vi "Autorange path verification.vi"() -> ()   [LabVIEW 2016]
uses:
  <instrlib>/Zurich Instruments LabOne/Public/ziTypeHandle.ctl
  <vilib>/regexp/Match Regular Expression.xnode
  <instrlib>/Zurich Instruments LabOne/Zurich Instruments LabOne.lvlib
panel:
  out "Path Out":string
  out "Handle Out":T1 {"Handle" format="0x%08x"; "Conn" format="0x%08x"}
  in  "Handle In":T1 {"Handle" format="0x%08x"; "Conn" format="0x%08x"}
  out "concatenated string":string
  out "x >= 0?":bool
  in  "Path 3":string="sigins/0/autorange"
  out "Coerced to new path":string
  in  "Path 2":string="sigins/0/autorange"
  in  "error in (no error) 2":errorcluster
  out "error out 2":errorcluster
  out "error out":errorcluster
  in  "error in (no error)":errorcluster
  in  "Path":string="sigins/0/autorange"
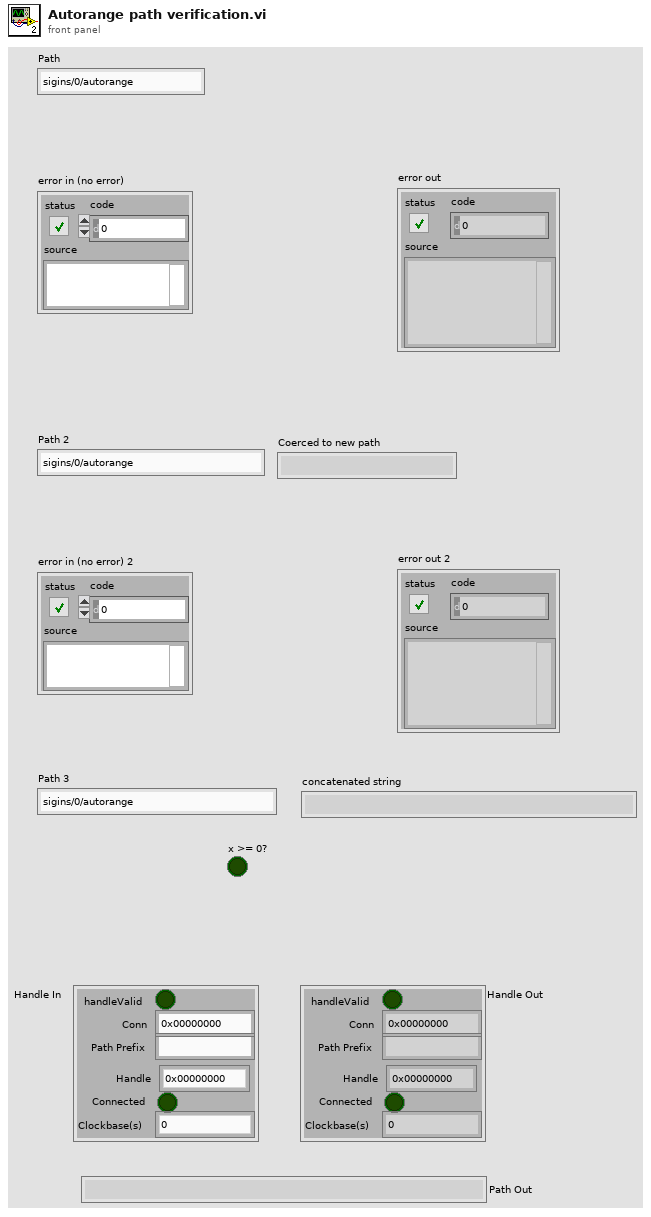
[diagram p1: front panel]
types:
  T1 = typedef "Zurich Instruments LabOne.lvlib/ziTypeHandle.ctl" = cluster{"handleValid":bool, "Conn":u64, "Path Prefix":string, "Handle":u64, "Connected":bool, "Clockbase(s)":dbl}
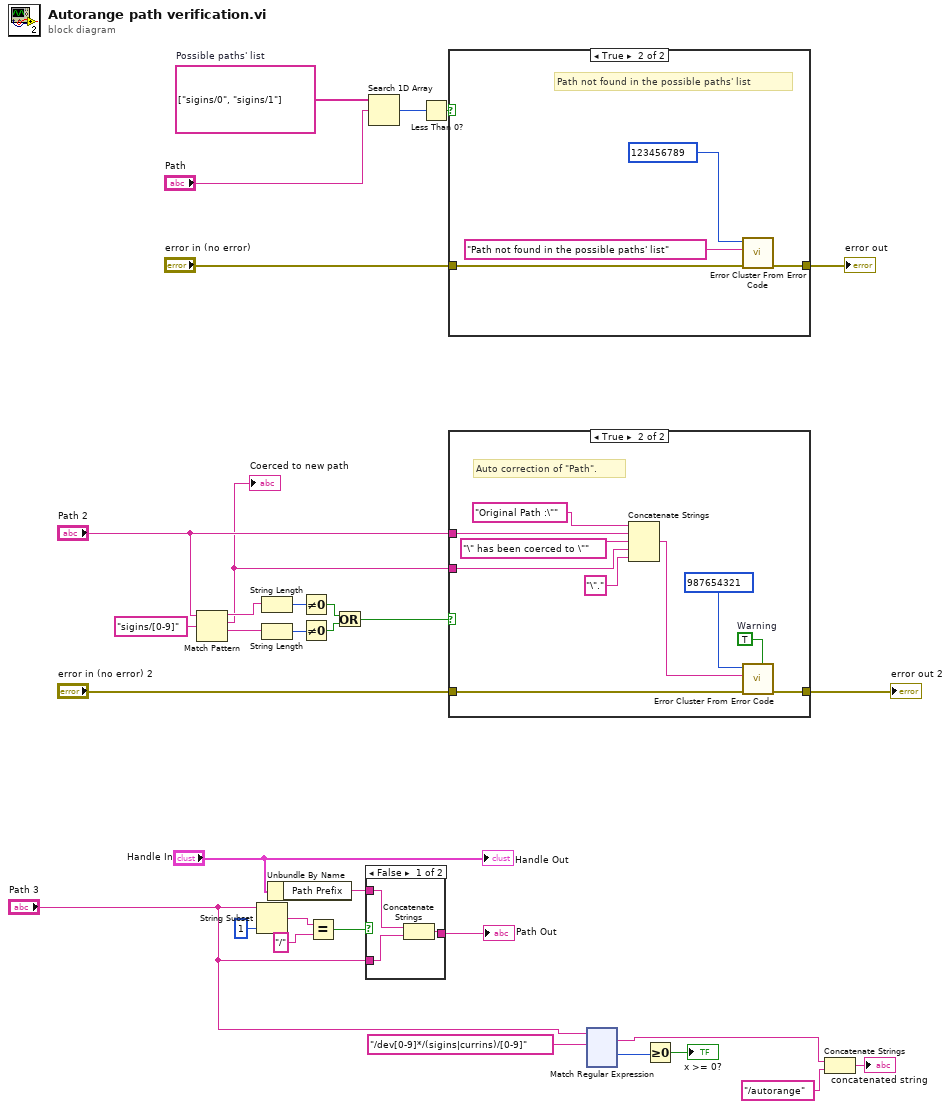
[diagram p0: block diagram]
diagram:
  w32 = string[] ["sigins/0", "sigins/1"]  # Possible paths' list
  n1 = Match Pattern(string="Path 2", regular expression="sigins/[0-9]") -> (before substring=w23:string, match substring=w16:string, after substring=w24:string)  [unwired: 1 in, 1 out]
  "Coerced to new path" <- w16
  n2 = String Subset(string="Path 3", length (rest)=1 ("length (rest)")) -> (substring=w7:string)  [unwired: 1 out]
  n3 = String Length(string=w23) -> (length=w22:i32)
  n4 = String Length(string=w24) -> (length=w21:i32)
  n5 = Unbundle By Name("Handle In") -> ("Path Prefix"=w5:string)
  n6 = Not Equal To 0?(x=w22) -> (x != 0?=w19:bool)
  n7 = Not Equal To 0?(x=w21) -> (x != 0?=w20:bool)
  n8 = Equal?(x=w7, y="/") -> (x = y?=w9:bool)
  n9 = Or(x=w19, y=w20) -> (x .or. y?=w18:bool)
  n10 = case shown="False" w9 {
    tunnel: w5 -> [w33 _]
    tunnel: [w35 w36] -> w3
    tunnel: "Path 3" -> [w34 w36]
    frame False {
      n11 = Concatenate Strings(w33, w34) -> (w35:string)
    }
    frame True {
    }
  }
  "Path Out" <- w3
  n12 = Search 1D Array(1D array=w32, element="Path") -> (index of element=w30:i32)  [unwired: 1 in]
  n13 = Less Than 0?(x=w30) -> (x < 0?=w29:bool)
  n14 = case shown="True" w29 {
    tunnel: "error in (no error)" -> [w37 w41]
    tunnel: [w37 w40] -> w27
    frame False {
    }
    frame True {
      # "Path not found in the possible paths' list"
      n15 = call <vilib>:"Error Cluster From Error Code.vi"("error in (no error)"=w41, "error message (\"\")"="Path not found in the possible paths' list" ("error message (\"\")"), "error code (0)"=123456789) -> ("error out"=w40:errorcluster)  [unwired: 6 in]
    }
  }
  "error out" <- w27
  n16 = case shown="True" w18 {
    tunnel: "error in (no error) 2" -> [w42 w52]
    tunnel: [w42 w51] -> w12
    tunnel: "Path 2" -> [_ w47]
    tunnel: w16 -> [_ w45]
    frame False {
    }
    frame True {
      w49 = TRUE  # Warning
      # "Auto correction of \"Path\"."
      n17 = Concatenate Strings("Original Path :\"", w47, "\" has been coerced to \"" ("string"), w45, "\"." ("string")) -> (w43:string)
      n18 = call <vilib>:"Error Cluster From Error Code.vi"("is warning? (False)"=w49, "error in (no error)"=w52, "error message (\"\")"=w43, "error code (0)"=987654321) -> ("error out"=w51:errorcluster)  [unwired: 5 in]
    }
  }
  "error out 2" <- w12
  n19 = xnode "Match Regular Expression"("input string"="Path 3", "regular expression"="/dev[0-9]*/(sigins|currins)/[0-9]") -> ("whole match"=w1:string, "offset past match"=w14:i32)  [unwired: 4 in, 3 out]
  n20 = Greater Or Equal To 0?(x=w14) -> (x >= 0?=→"x >= 0?":bool)
  n21 = Concatenate Strings(w1, "/autorange") -> (→"concatenated string":string)
  "Handle Out" <- "Handle In"
